vi "waveform gen_DC.vi"(1 "Scale factor":u16=1, 2 "Boolean":bool, 3 "Exposure Time (s)":dbl(ring)=0.5 items=["0.2"=0.2, "0.5"=0.5, "1.0"=1.0, "4.0"=4.0, "8.0"=8.0], 4 "Laser Power%(0-100)":dbl=10.0) -> (0 "waveform":waveform(dbl)[](array[waveform]))   [LabVIEW 2018]
uses:
  <vilib>/Analysis/coordinate.llb/2D Cartesian Coordinate Rotation (Array).vi
  <vilib>/measure/NI_MABase.lvlib
  <vilib>/Analysis/NI_AALPro.lvlib
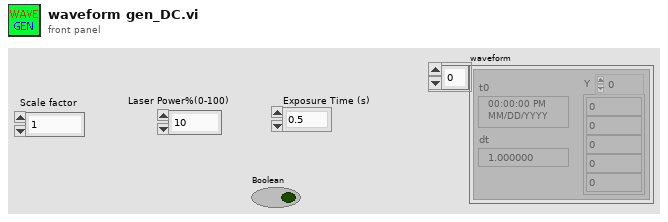
[diagram p1: front panel]
types:
  T1 = cluster{"Galvo/Pockels Cell Sampling Info":dbl, "#s":dbl}
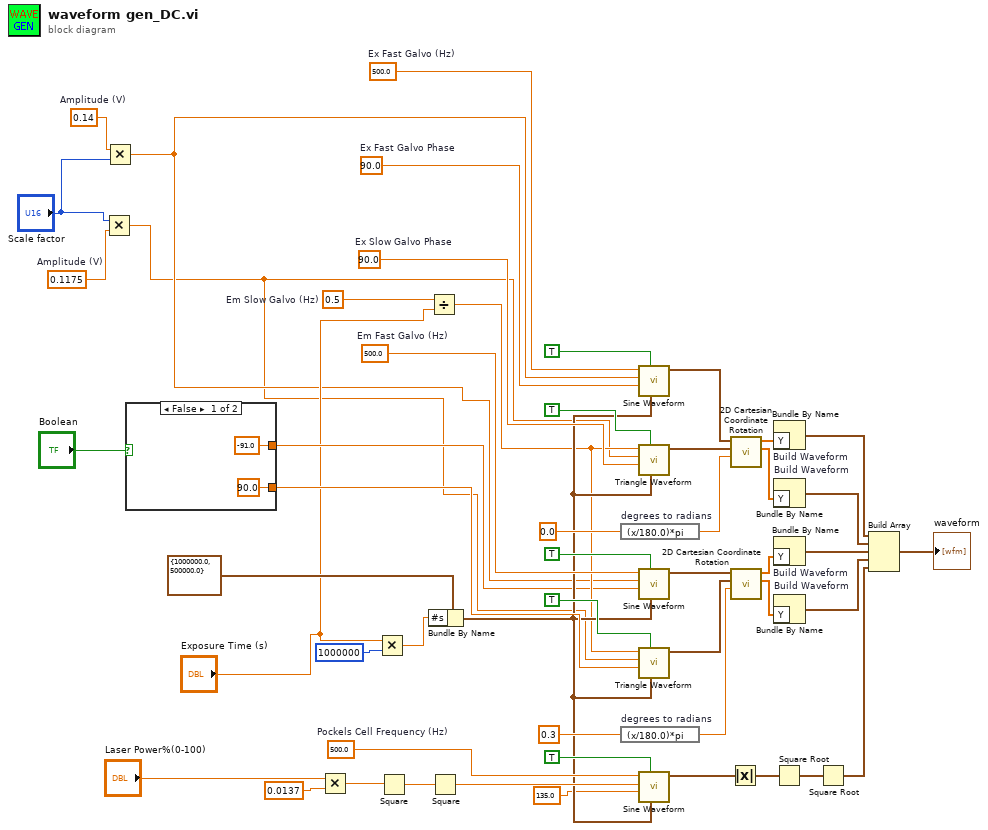
[diagram p0: block diagram]
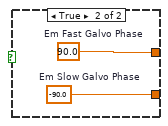
[diagram p2: hidden frame]
diagram:
  w13 = 0.5  # Em Slow Galvo (Hz)
  w2 = 0.1175  # Amplitude (V)
  w51 = 500.0  # Ex Fast Galvo (Hz)
  w5 = 0.14  # Amplitude (V)
  w50 = 500.0  # Pockels Cell Frequency (Hz)
  w48 = 500.0  # Em Fast Galvo (Hz)
  w44 = 90.0  # Ex Slow Galvo Phase
  w45 = 90.0  # Ex Fast Galvo Phase
  n1 = Multiply(x="Scale factor", y=w2) -> (x*y=w1:dbl)
  n2 = Multiply(x=w5, y="Scale factor") -> (x*y=w4:dbl)
  n3 = case shown="False" "Boolean" {
    tunnel: [90.0 ("Em Slow Galvo Phase") w56] -> w18
    tunnel: [-91.0 ("Em Fast Galvo Phase") w55] -> w10
    frame False {
    }
    frame True {
      w55 = 90.0  # Em Fast Galvo Phase
      w56 = -90.0  # Em Slow Galvo Phase
    }
  }
  n4 = Multiply(x="Laser Power%(0-100)", y=0.0137 ("data")) -> (x*y=w49:dbl)
  n5 = Multiply(x="Exposure Time (s)", y=1000000) -> (x*y=w14:dbl)
  n6 = Square(x=w49) -> (x^2=w37:dbl)
  n7 = Divide(x=w13, y="Exposure Time (s)") -> (x/y=w12:dbl)
  n8 = Bundle By Name(cluster=T1 {"Galvo/Pockels Cell Sampling Info"=1000000.0, "#s"=500000.0} ("Sampling Info"), "#s"=w14) -> (w16:T1)
  n9 = Square(x=w37) -> (x^2=w36:dbl)
  n10 = expression code="(x/180.0)*pi" "degrees to radians"(0.0 ("Ex Theta")) -> (w22:dbl)
  n11 = expression code="(x/180.0)*pi" "degrees to radians"(0.3 ("Em Theta")) -> (w19:dbl)
  n12 = call <vilib>:"Sine Waveform.vi"("sampling info"=w16, "reset signal"=TRUE, "phase"=w45, "amplitude"=w4, "frequency"=w51) -> ("signal out"=w34:waveform(dbl))  [unwired: 5 in, 1 out]
  n13 = call <vilib>:"Triangle Waveform.vi"("sampling info"=w16, "reset signal"=TRUE, "phase"=w44, "amplitude"=w1, "frequency"=w12) -> ("signal out"=w35:waveform(dbl))  [unwired: 5 in, 1 out]
  n14 = call <vilib>:"Sine Waveform.vi"("sampling info"=w16, "reset signal"=TRUE, "phase"=w10, "amplitude"=w4, "frequency"=w48) -> ("signal out"=w21:waveform(dbl))  [unwired: 5 in, 1 out]
  n15 = call <vilib>:"Triangle Waveform.vi"("sampling info"=w16, "reset signal"=TRUE, "phase"=w18, "amplitude"=w1, "frequency"=w12) -> ("signal out"=w26:waveform(dbl))  [unwired: 5 in, 1 out]
  n16 = call <vilib>:"Sine Waveform.vi"("sampling info"=w16, "reset signal"=TRUE, "phase"=135.0, "amplitude"=w36, "frequency"=w50) -> ("signal out"=w47:waveform(dbl))  [unwired: 5 in, 1 out]
  n17 = Absolute Value(x=w47) -> (abs(x)=w39:waveform(dbl))
  n18 = call-poly <vilib>:"2D Cartesian Coordinate Rotation.vi"("theta"=w22, "Y"=w35, "X"=w34) -> ("Y Out"=w31:dbl[], "X Out"=w33:dbl[])  [unwired: 6 in, 1 out]
  n19 = call-poly <vilib>:"2D Cartesian Coordinate Rotation.vi"("theta"=w19, "Y"=w26, "X"=w21) -> ("Y Out"=w27:dbl[], "X Out"=w28:dbl[])  [unwired: 6 in, 1 out]
  n20 = Bundle By Name "Build Waveform"("Y"=w33) -> (w32:waveform(dbl))  [unwired: 1 in]
  n21 = Bundle By Name "Build Waveform"("Y"=w31) -> (w30:waveform(dbl))  [unwired: 1 in]
  n22 = Bundle By Name "Build Waveform"("Y"=w28) -> (w24:waveform(dbl))  [unwired: 1 in]
  n23 = Bundle By Name "Build Waveform"("Y"=w27) -> (w25:waveform(dbl))  [unwired: 1 in]
  n24 = Square Root(x=w39) -> (sqrt(x)=w38:waveform(dbl))
  n25 = Square Root(x=w38) -> (sqrt(x)=w29:waveform(dbl))
  n26 = Build Array "Build Array"(w32, w30, w24, w25, w29) -> (→"waveform":waveform(dbl)[])
